vi "_interfacebrowser Filter Tree Data.vi"(9 "FilterOption":T2, 10 "Filter":string, 11 "TreeData":T1) -> (3 "TreeData 2":T1)   [LabVIEW 2017, in "interfacebrowser.lvlib"]
uses:
  interfacebrowser.lvlib
  _SubModules/Def-TreeData.ctl
  _SubModules/Def-FilterOption.ctl
  _csmHelper/API with lvcsm Support/CSM-Helper API with lvcsm Support.lvlib
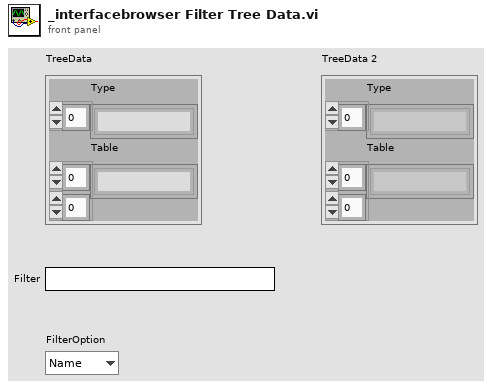
[diagram p1: front panel]
types:
  T1 = typedef "Def-TreeData.ctl" = cluster{"Type":string[], "Table":string[][]}
  T2 = typedef "Def-FilterOption.ctl" = enum16{"Name", "State"}
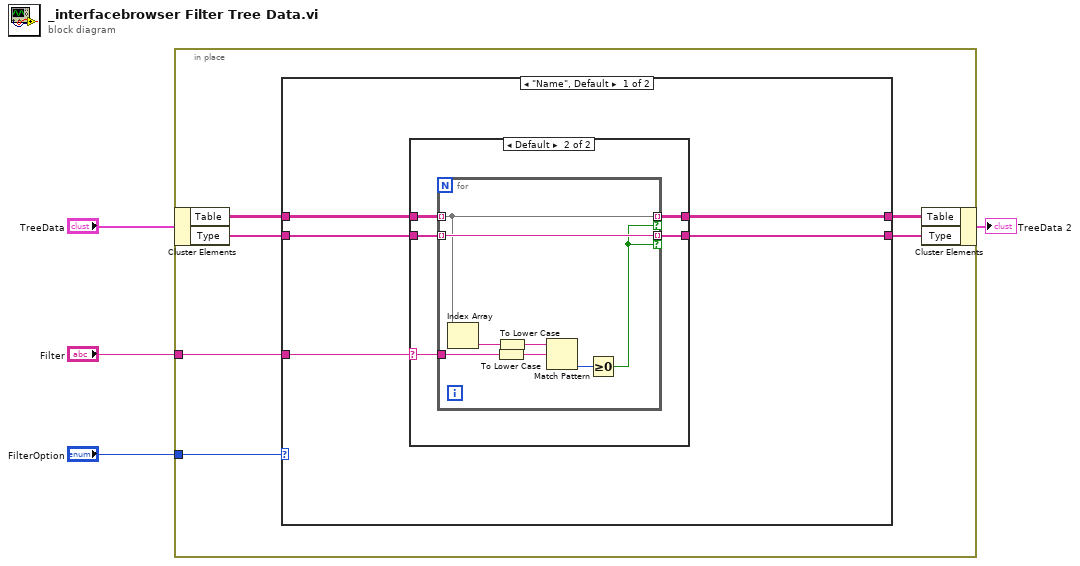
[diagram p0: block diagram]
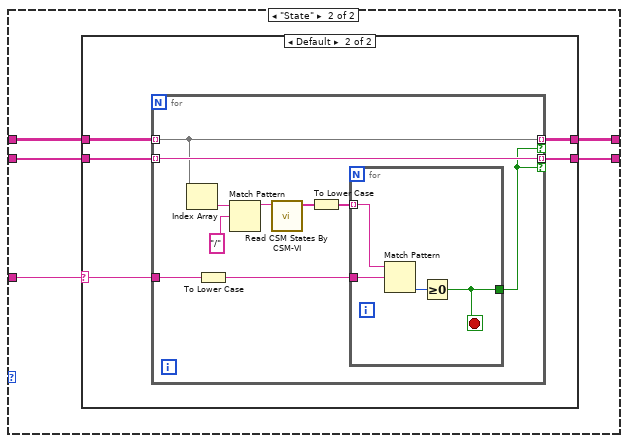
[diagram p3: hidden frame]
diagram:
  n1 = in-place {
    in-place-border: "Filter" -> [w10]
    in-place-border: "FilterOption" -> [w5]
    n2 = in-place-cluster #1("TreeData") -> ("Table"=w9:string[][], "Type"=w8:string[])
    n3 = case shown="\"Name\", Default" w5 {
      tunnel: w10 -> [w15 w35]
      tunnel: w9 -> [w14 w34]
      tunnel: w8 -> [w13 w33]
      tunnel: [w12 w32] -> w7
      tunnel: [w11 w31] -> w6
      frame "Name", Default {
        n4 = case shown="Default" w15 {
          selector: w15 -> [_ w21]
          tunnel: w14 -> [w17 w22]
          tunnel: [w16 w20] -> w11
          tunnel: w13 -> [w16 w19]
          tunnel: [w17 w18] -> w12
          frame "" {
          }
          frame Default {
            n5 = for {
              tunnel: w22 -> [w27] mode=indexing
              tunnel: w21 -> [w29]
              tunnel: [w28] -> w20 mode=indexing if=w25
              tunnel: w19 -> [w28] mode=indexing
              tunnel: [w27] -> w18 mode=indexing if=w25
              n6 = Index Array(array=w27) -> (element=w30:string)  [unwired: 1 in]
              n7 = To Lower Case(string=w29) -> (all lower case string=w23:string)
              n8 = To Lower Case(string=w30) -> (all lower case string=w24:string)
              n9 = Match Pattern(string=w24, regular expression=w23) -> (offset past match=w26:i32)  [unwired: 1 in, 3 out]
              n10 = Greater Or Equal To 0?(x=w26) -> (x >= 0?=w25:bool)
            }
          }
        }
      }
      frame "State" {
        n11 = case shown="\"\"" w35 {
          selector: w35 -> [_ w41]
          tunnel: w34 -> [w37 w42]
          tunnel: [w36 w40] -> w31
          tunnel: w33 -> [w36 w39]
          tunnel: [w37 w38] -> w32
          frame "" {
          }
          frame Default {
            n12 = for {
              tunnel: w42 -> [w48] mode=indexing
              tunnel: w41 -> [w52]
              tunnel: [w51] -> w40 mode=indexing if=w50
              tunnel: w39 -> [w51] mode=indexing
              tunnel: [w48] -> w38 mode=indexing if=w50
              n13 = Index Array(array=w48) -> (element=w47:string)  [unwired: 1 in]
              n14 = To Lower Case(string=w52) -> (all lower case string=w49:string)
              n15 = Match Pattern(string=w47, regular expression="/") -> (before substring=w45:string)  [unwired: 1 in, 3 out]
              n16 = call "Read CSM States By CSM-VI.vi"("CSM VI"=w45) -> ("Array"=w44:string[])  [unwired: 9 in, 1 out]
              n17 = To Lower Case(string=w44) -> (all lower case string=w43:string[])
              n18 = for {
                tunnel: [w53] -> w50
                tunnel: w49 -> [w55]
                tunnel: w43 -> [w54] mode=indexing
                stop <- w53 stop-if-true
                n19 = Match Pattern(string=w54, regular expression=w55) -> (offset past match=w56:i32)  [unwired: 1 in, 3 out]
                n20 = Greater Or Equal To 0?(x=w56) -> (x >= 0?=w53:bool)
              }
            }
          }
        }
      }
    }
    n21 = in-place-cluster #1("Table"=w7, "Type"=w6) -> (→"TreeData 2":T1)
  }
